vi "Hardware In - NI 9220-1 (AI).vi"(11 "FPGA Ref":T1) -> (3 "9220-1":T2)   [LabVIEW 2015, in "ECS-RT.lvlib"]
uses:
  ECS-RT.lvlib
  Typedefs/Raw Inputs/NI9220.ctl
  Typedefs/FPGA Refs/Generic FPGA Ref.ctl
  <vilib>/rvi/errors/niLvFpgaAdjustHostInterfaceError.vi
  <vilib>/Utility/error.llb/Error Cluster From Error Code.vi
  <vilib>/rvi/interface/nirviReadWriteControl/nirviReadWriteControl.xnode
  <vilib>/rvi/interface/Simulation/niFpgaSimulationCallBeginRW.vi
  NiFpgaLv.dll
  ECS-Shared.lvlib
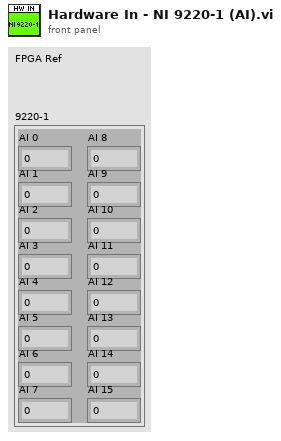
[diagram p1: front panel]
types:
  T1 = typedef "ECS-Shared.lvlib/Generic FPGA Ref.ctl" = refnum<k20>
  T2 = typedef "ECS-Shared.lvlib/NI9220.ctl" = cluster{"AI 0":sgl, "AI 1":sgl, "AI 2":sgl, "AI 3":sgl, "AI 4":sgl, "AI 5":sgl, "AI 6":sgl, "AI 7":sgl, "AI 8":sgl, "AI 9":sgl, "AI 10":sgl, "AI 11":sgl, "AI 12":sgl, "AI 13":sgl, "AI 14":sgl, "AI 15":sgl}
  T3 = cluster{"[0]":sgl, "[1]":sgl, "[2]":sgl, "[3]":sgl, "[4]":sgl, "[5]":sgl, "[6]":sgl, "[7]":sgl, "[8]":sgl, "[9]":sgl, "[10]":sgl, "[11]":sgl, "[12]":sgl, "[13]":sgl, "[14]":sgl, "[15]":sgl}
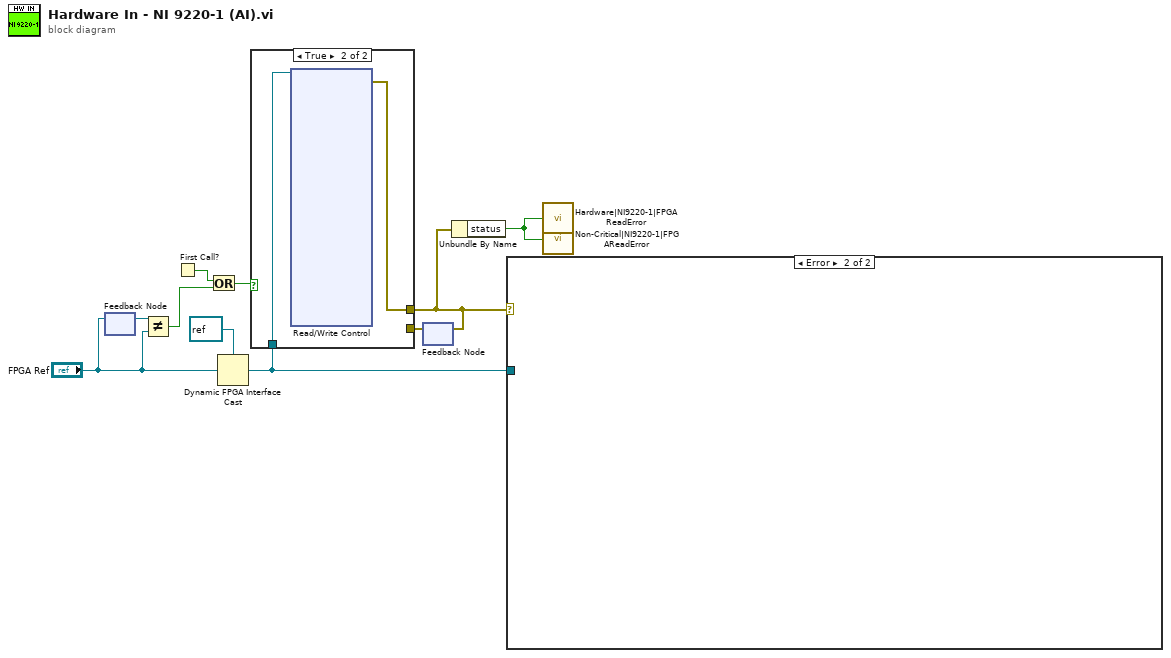
[diagram p0: block diagram]
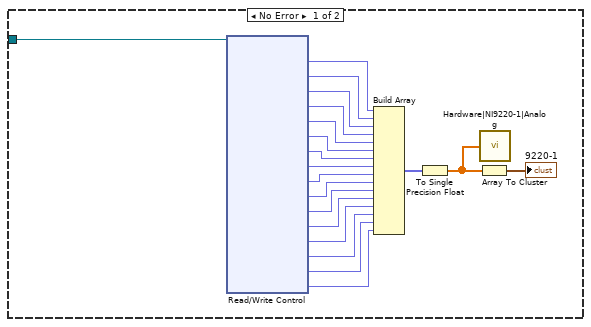
[diagram p3: hidden frame]
diagram:
  n1 = feedback #1() -> (w9:T1)  [unwired: 1 in]
  n2 = feedback-in #1("FPGA Ref") -> ()
  n3 = Not Equal?(x=w9, y="FPGA Ref") -> (x != y?=w10:bool)
  n4 = First Call?() -> (First Call?: T/F=w8:bool)
  n5 = Or(x=w8, y=w10) -> (x .or. y?=w7:bool)
  n6 = Dynamic FPGA Interface Cast(Session In=refnum<k20> refnum ("FPGA VI Reference Out"), Type="FPGA Ref") -> (Session Out=w4:refnum<k20>)
  n7 = feedback #2() -> (w6:errorcluster)  [unwired: 1 in]
  n8 = case shown="True" w7 {
    tunnel: [w11 w13] -> w2
    tunnel: w6 -> [w11 _]
    tunnel: w4 -> [_ w12]
    frame False {
    }
    frame True {
      n9 = xnode "Read/Write Control"("FPGA VI Reference In"=w12) -> ("error out"=w13:errorcluster)  [unwired: 1 in, 17 out]
    }
  }
  n10 = feedback-in #2(w2) -> ()
  n11 = Unbundle By Name(w2) -> ("status"=w1:bool)
  n12 = case shown="Error" w2 {
    tunnel: w4 -> [w33 _]
    frame No Error {
      n13 = xnode "Read/Write Control"("FPGA VI Reference In"=w33) -> ("9220-1/AI0"=w32:fxp<+/-,24,5>, "9220-1/AI1"=w31:fxp<+/-,24,5>, "9220-1/AI2"=w30:fxp<+/-,24,5>, "9220-1/AI3"=w29:fxp<+/-,24,5>, "9220-1/AI4"=w28:fxp<+/-,24,5>, "9220-1/AI5"=w27:fxp<+/-,24,5>, "9220-1/AI6"=w26:fxp<+/-,24,5>, "9220-1/AI7"=w25:fxp<+/-,24,5>, "9220-1/AI8"=w24:fxp<+/-,24,5>, "9220-1/AI9"=w23:fxp<+/-,24,5>, "9220-1/AI10"=w22:fxp<+/-,24,5>, "9220-1/AI11"=w21:fxp<+/-,24,5>, "9220-1/AI12"=w20:fxp<+/-,24,5>, "9220-1/AI13"=w19:fxp<+/-,24,5>, "9220-1/AI14"=w18:fxp<+/-,24,5>, "9220-1/AI15"=w17:fxp<+/-,24,5>)  [unwired: 1 in, 2 out]
      n14 = Build Array(w32, w31, w30, w29, w28, w27, w26, w25, w24, w23, w22, w21, w20, w19, w18, w17) -> (w16:fxp<+/-,24,5>[])
      n15 = To Single Precision Float(number=w16) -> (single precision float=w15:sgl[])
      n16 = Array To Cluster(array=w15) -> (cluster=→"9220-1":T3)
      n17 = call "Hardware|NI9220-1|Analog"("Value"=w15) -> ()
    }
    frame Error {
    }
  }
  n18 = call "Hardware|NI9220-1|FPGAReadError"("Value"=w1) -> ()
  n19 = call "Non-Critical|NI9220-1|FPGAReadError"("Fault"=w1) -> ()  [unwired: 2 in]
